vi "试件参数.vi"() -> (0 "error out":errorcluster caption="错误输出")   [LabVIEW 2016]
panel:
  in  "读取按钮":bool
  in  "取消按钮":bool
  in  "确定按钮":bool
  in  "横截面积(mm^2)":dbl
  in  "试件长度(mm)":dbl
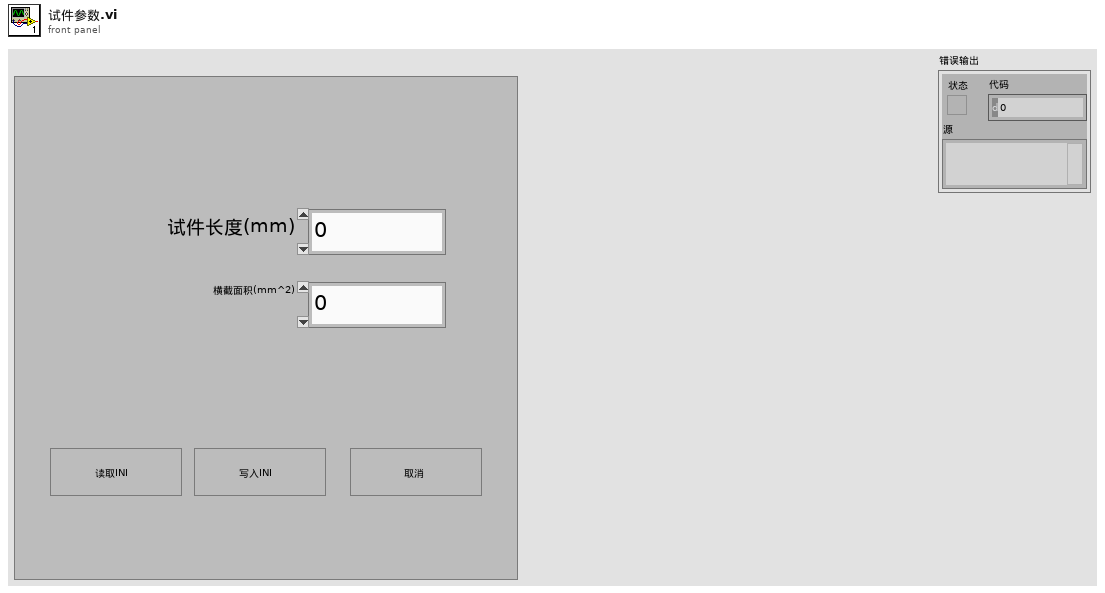
[diagram p1: front panel]
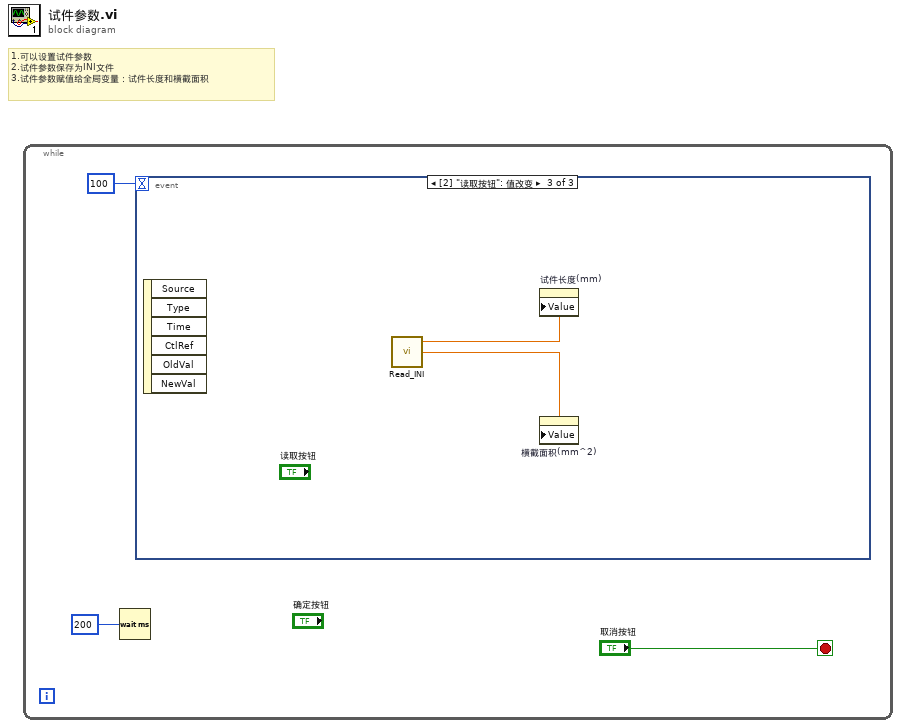
[diagram p0: block diagram]
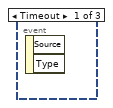
[diagram p2: hidden frame]
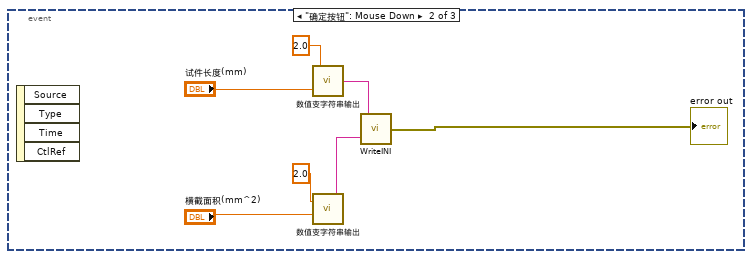
[diagram p3: hidden frame]
diagram:
  # "1.可以设置试件参数\n2.试件参数保存为INI文件\n3.试件参数赋值给全局变量：试件长度和横截面积"
  n1 = while {
    stop <- "取消按钮" stop-if-true
    n2 = Wait (ms)(milliseconds to wait=u32 200 ("等待时间（毫秒）")) -> ()  [unwired: 1 out]
    n3 = event shown="[2] \"读取按钮\": 值改变" {
      selector: _ -> [_ _ _]
      dyn-events: _ -> [_ _ _]
      timeout: 100 -> [_ _ _]
      event Timeout {
        n4 = event-data() -> ()  [unwired: 1 in, 2 out]
      }
      event "确定按钮": Mouse Down {
        n5 = event-data() -> ()  [unwired: 1 in, 4 out]
        n6 = call "数值变字符串输出.vi"("浮点数值"="试件长度(mm)", "小数点"=2.0) -> ("输出字符串"=w9:string)
        n7 = call "数值变字符串输出.vi"("浮点数值"="横截面积(mm^2)", "小数点"=2.0) -> ("输出字符串"=w5:string)
        n8 = call "WriteINI.vi"("试件面积"=w5, "试件长度"=w9) -> ("error out"=→"error out":errorcluster)
      }
      event "读取按钮": Value Change {
        n9 = event-data() -> ()  [unwired: 1 in, 6 out]
        n10 = call "Read_INI.vi"() -> ("试件面积"=w11:dbl, "试件长度"=w12:dbl)  [unwired: 1 out]
        n11 = property on="试件长度(mm)" class="DigNum (严格)"("Value"=w12) -> ()  [unwired: 2 in, 2 out]
        n12 = property on="横截面积(mm^2)" class="DigNum (严格)"("Value"=w11) -> ()  [unwired: 2 in, 2 out]
      }
    }
  }
